vi "Initialize Multi Listbox ItemName.vi"(8 "error in (no error)":errorcluster, 11 "Multicolumn Listbox In":refnum<vi>) -> (0 "error out":errorcluster, 3 "Multicolumn Listbox Out":refnum<vi>)   [LabVIEW 2012]
uses:
  Custom Type/Row and Col Option.ctl
  ListBox/Custom Type/Read and Write Mode.ctl
  Property/Set and Get Num of Rows Or Cols.vi
  Property/Set and Get ItemNames.vi
  Mlistbox Tools.lvlib
  ListBox/Listbox Tool.lvlib
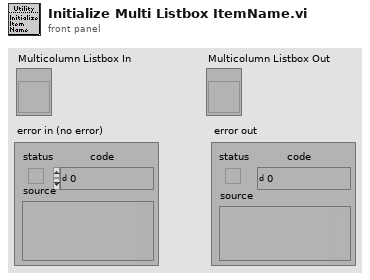
[diagram p1: front panel]
types:
  T1 = typedef "Listbox Tool.lvlib/Read and Write Mode.ctl" = enum16{"Read", "Write"}
  T2 = typedef "Mlistbox Tools.lvlib/Row and Col Option.ctl" = enum16{"Row", "Col"}
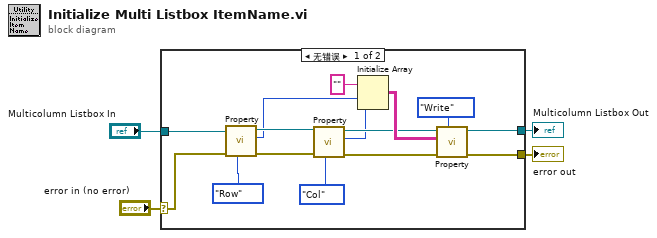
[diagram p0: block diagram]
diagram:
  n1 = case shown="无错误" "error in (no error)" {
    selector: "error in (no error)" -> [w18 w20]
    tunnel: [w8 w20] -> w3
    tunnel: "Multicolumn Listbox In" -> [w17 _]
    tunnel: [w9 _] -> w1
    frame No Error {
      n2 = call-poly "Property.vi"("Row Or Col"=Row_and_Col_Option."Row", "错误输入"=w18, "Mlistbox Ref"=w17) -> ("错误输出"=w14:errorcluster, "Number of Rows or Cols Out"=w6:u32, "Mlistbox Ref Dup"=w15:refnum<vi>)  [unwired: 6 in]
      n3 = call-poly "Property.vi"("Row Or Col"=Row_and_Col_Option."Col", "错误输入"=w14, "Mlistbox Ref"=w15) -> ("错误输出"=w12:errorcluster, "Number of Rows or Cols Out"=w5:u32, "Mlistbox Ref Dup"=w10:refnum<vi>)  [unwired: 6 in]
      n4 = Initialize Array("", w6, w5) -> (w11:string[][])
      n5 = call-poly "Property.vi"("Mode"=Read_and_Write_Mode."Write", "错误输入"=w12, "ItemNames In"=w11, "Mlistbox Ref"=w10) -> ("错误输出"=w8:errorcluster, "Mlistbox Ref Dup"=w9:refnum<vi>)  [unwired: 5 in, 1 out]
    }
    frame Error {
    }
  }
  "error out" <- w3
  "Multicolumn Listbox Out" <- w1
